vi "valve_visa_test.vi"() -> ()   [LabVIEW 2013]
uses:
  <vilib>/Instr/_visa.llb/VISA Configure Serial Port (Instr).vi
panel:
  out "read buffer":string
  in  "Command option":string
  in  "COMMANDS":T1(ring)
  out "error out 3":errorcluster
  out "error out 2":errorcluster
  out "Error OUT":errorcluster
  out "error out":errorcluster
  in  "error in (no error)":errorcluster
  in  "VISA resource name":refnum<visa-resource-name>="COM1"
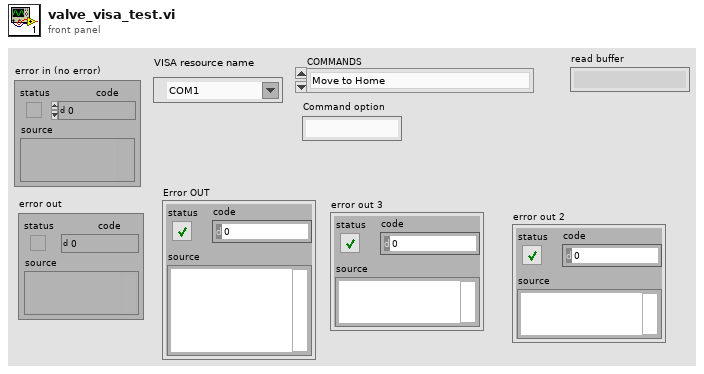
[diagram p1: front panel]
types:
  T1 = enum16{"Move to Home", "Set Positions", "Set Actuator Mode", "OTHER", "Set Direction", "CW Move", "CCW Move"}
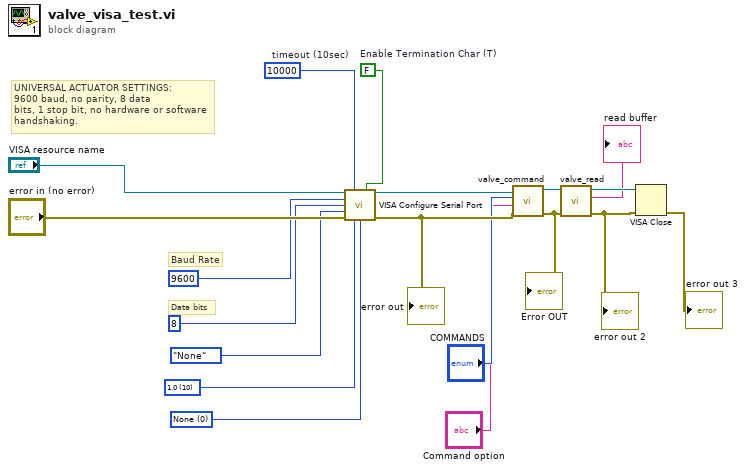
[diagram p0: block diagram]
diagram:
  w12 = u16 0 items=["None", "XON/XOFF", "RTS/CTS", "XON/XOFF & RTS/CTS", "DTR/DSR", "XON/XOFF & DTR/DSR"] ("flow control (0:none)")
  w13 = u16 10 items=["1.0"=10, "1.5"=15, "2.0"=20] ("stop bits (10: 1 bit)")
  w11 = FALSE  # Enable Termination Char (T)
  w18 = u32 10000  # timeout (10sec)
  # "UNIVERSAL ACTUATOR SETTINGS:\n9600 baud, no parity, 8 data \nbits, 1 stop bit, no hardware or software \nhandshaking."
  # "Data bits"
  # "Baud Rate"
  n1 = call-poly "VISA Configure Serial Port"("VISA resource name"="VISA resource name", "timeout (10sec)"=w18, "Enable Termination\nChar (T)"=w11, "baud rate (9600)"=u32 9600, "data bits (8)"=u16 8, "parity (0:none)"=enum16{"None", "Odd", "Even", "Mark", "Space"}."None", "error in (no error)"="error in (no error)", "stop bits (10: 1 bit)"=w13, "flow control (0:none)"=w12) -> ("VISA resource name out"=w8:refnum<visa-resource-name>, "error out"=w9:errorcluster)  [unwired: 5 in]
  "error out" <- w9
  n2 = call "valve_command.vi"("Error IN"=w9, "Command option"="Command option", "COMMANDS"="COMMANDS", "VISA Resource IN"=w8) -> ("Error OUT"=w7:errorcluster, "Visa Resource OUT"=w10:refnum<visa-resource-name>)  [unwired: 6 in]
  "Error OUT" <- w7
  n3 = call "valve_read.vi"("error in (no error)"=w7, "reference"=w10) -> ("error out"=w5:errorcluster, "read buffer"=→"read buffer":string, "VISA resource name out"=w6:refnum<visa-resource-name>)  [unwired: 7 in]
  "error out 2" <- w5
  n4 = VISA Close(VISA resource name=w6, error in (no error)=w5) -> (error out=→"error out 3":errorcluster)
